vi "configure operation.vi"(7 "EthernetIP configuration":refnum<class "EthernetIP configuration.lvclass">, 8 "error in":errorcluster, 10 "line item in":T1, 11 "engine configuration in":refnum<class "engine configuration.lvclass">) -> (0 "error out":errorcluster, 1 "success":bool, 2 "line item out":T1, 5 "changed":bool)   [LabVIEW 2013, in "EthernetIP editor node.lvclass"]
uses:
  EthernetIP editor node.lvclass
  table line.ctl
  <vilib>/NI/TBM Modules/Ethernet IP/channel/EthernetIP Channel.lvclass
  <vilib>/NI/Module Execution Interface/Engine Configuration/engine configuration.lvclass
  <vilib>/NI/TBM Modules/Ethernet IP/configuration/EthernetIP configuration.lvclass
  <vilib>/NI/TBM Modules/Ethernet IP/configuration/EthernetIP configuration.lvclass/EthernetIP configuration.ctl
  <vilib>/NI/Tag Bus Module Framework/root configuration/TBM configuration.lvclass/TBM configuration.ctl
  <vilib>/NI/Tag Bus/tag/tag descriptor.lvclass/tag descriptor.ctl
  <vilib>/NI/TBM Modules/Ethernet IP/channel/EthernetIP Channel.lvclass/EthernetIP Channel.ctl
  <vilib>/NI/Tag Bus/tag/Data Type.ctl
  <vilib>/NI/Tag Bus Module Framework/channel/TBM channel.lvclass/TBM channel.ctl
  <vilib>/NI/TBM Modules/Ethernet IP/configuration/Read assemblies.vi
  <vilib>/NI/Tag Bus Module Framework/root configuration/Read instance name.vi
  <vilib>/NI/Tag Bus Module Framework/channel/Read channel classification.vi
  <vilib>/NI/Tag Bus/tag/read tag name.vi
  <vilib>/NI/Tag Bus/tag/read data type.vi
  <vilib>/NI/TBM Modules/Ethernet IP/channel/Read byte index.vi
  <vilib>/NI/TBM Modules/Ethernet IP/channel/Read subindex.vi
  <vilib>/NI/TBM Modules/Ethernet IP/channel/Read Instance ID.vi
  <vilib>/NI/Tag Bus/tag/write tag name.vi
  <vilib>/NI/Tag Bus/tag/write data type.vi
  <vilib>/NI/TBM Modules/Ethernet IP/channel/Write Instance ID.vi
  <vilib>/NI/Tag Bus Module Framework/channel/Write channel classification.vi
  <vilib>/NI/TBM Modules/Ethernet IP/channel/Write byte index.vi
  <vilib>/NI/TBM Modules/Ethernet IP/channel/Write subindex.vi
  <vilib>/NI/Tag Bus Module Framework/root configuration/create GUID.vi
  <vilib>/NI/Tag Bus/tag/tag descriptor.lvclass
panel:
  in  "refresh tags":bool
  in  "Tag":i32(listbox)
  in  "Type":i32(listbox)
  in  "Instance":i32(listbox)
  out "problem":string
  in  "subindex":i32 min=0 max=7 step=1
  in  "byte index":i32
  in  "Channel Name":string
  in  "cancel":bool
  in  "ok":bool
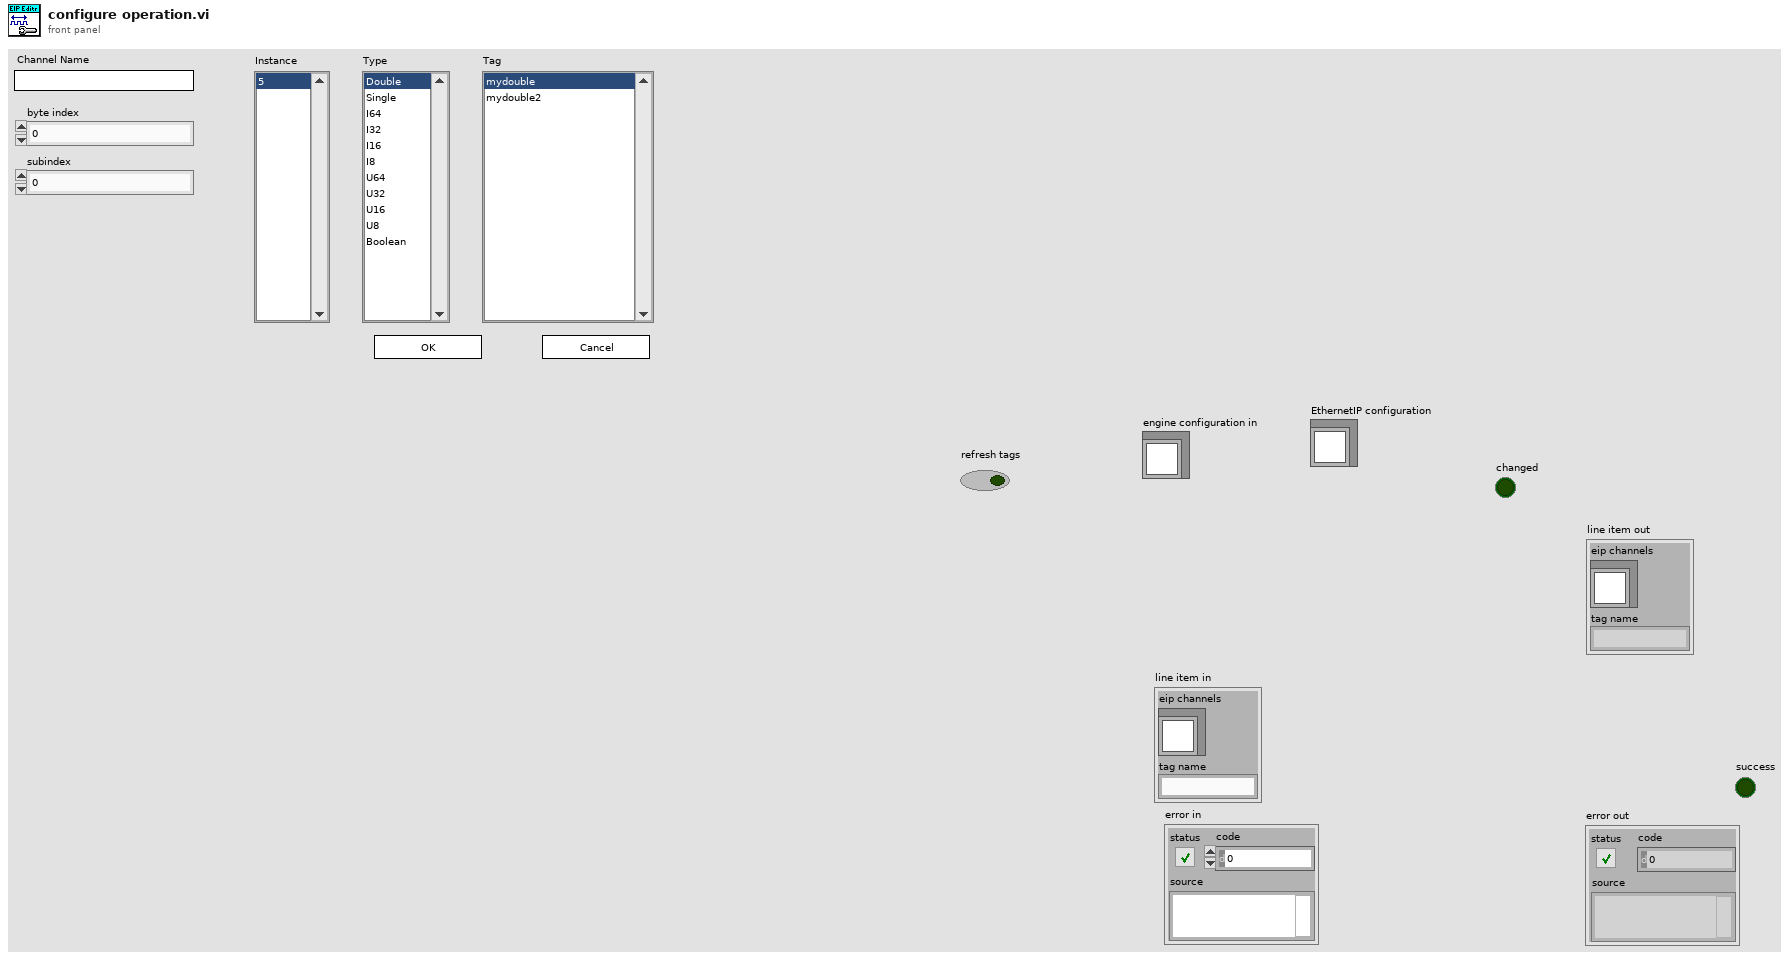
[diagram p1: front panel]
types:
  T1 = typedef "EthernetIP editor node.lvclass/table line.ctl" = cluster{"eip channels":refnum<class "EthernetIP Channel.lvclass">, "tag name":string}
  T2 = enum32{"Invalid", "Standard", "Closed", "Hidden", "Minimized", "Maximized"}
  T3 = enum32{"Invalid", "Default", "Floating", "Floating/Auto-Hide", "Modal"}
  T4 = enum8{"Enabled", "Disabled", "Disabled and Grayed Out"}
  T5 = typedef "tag bus.lvlib/tag descriptor.lvclass/Data Type.ctl" = enum16{"Double", "Single", "I64", "I32", "I16", "I8", "U64", "U32", "U16", "U8", "Boolean", "String", "Array of Double", "Array of Single", "Array of I64", "Array of I32", "Array of I16", "Array of I8", "Array of U64", "Array of U32", "Array of U16", "Array of U8", "Array of Boolean", "Array of String"}
  T6 = typedef "EthernetIP configuration.lvclass/assembly definition.ctl" = cluster{"name":string, "Instance ID":u32, "Type":T7, "Size (bytes)":u32}
  T7 = typedef "EthernetIP configuration.lvclass/assembly type.ctl" = enum32{"Producing", "Consuming"}
  T8 = enum32{"invalid app kind", "Development System", "Run Time System", "Student Edition", "Embedded LabVIEW", "Evaluation", "Custom"}
  T9 = typedef "TBM channel.lvclass/channel classification.ctl" = enum16{"input data", "output data", "processing parameter", "processing result"}
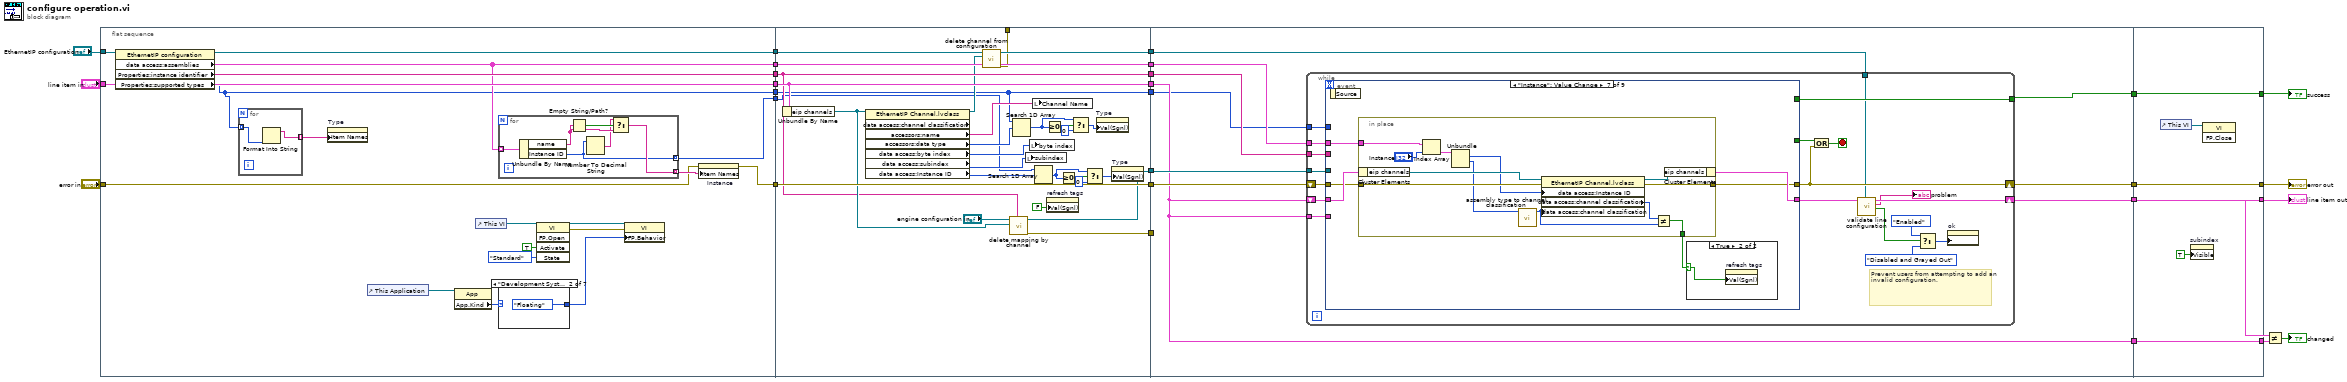
[diagram p0: block diagram]
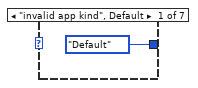
[diagram p2: hidden frame]
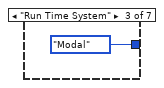
[diagram p3: hidden frame]
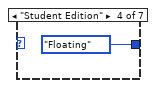
[diagram p4: hidden frame]
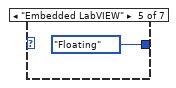
[diagram p5: hidden frame]
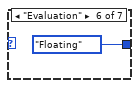
[diagram p6: hidden frame]
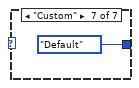
[diagram p7: hidden frame]
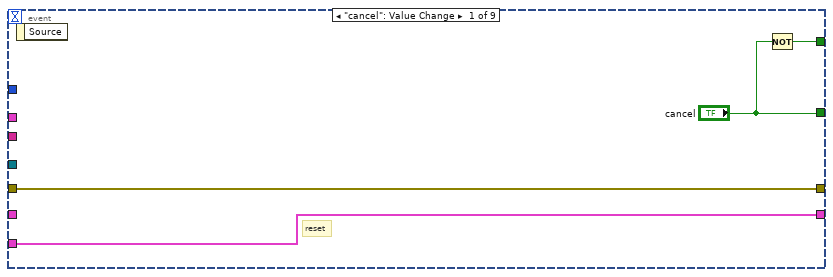
[diagram p8: hidden frame]
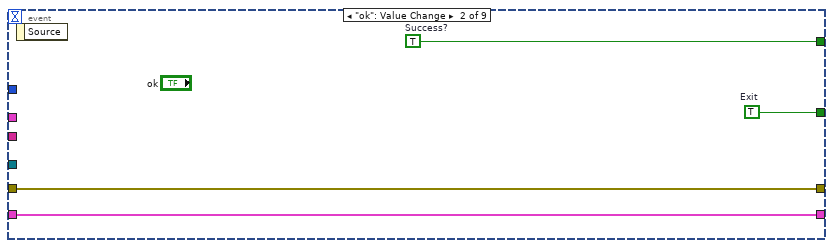
[diagram p9: hidden frame]
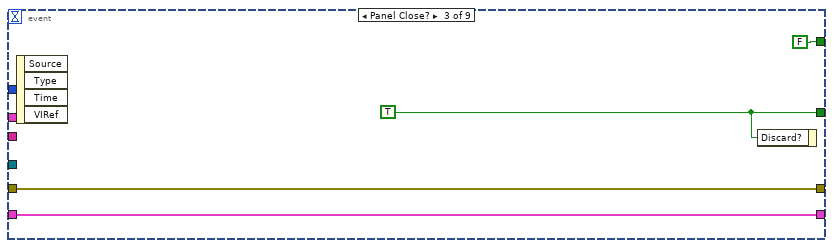
[diagram p10: hidden frame]
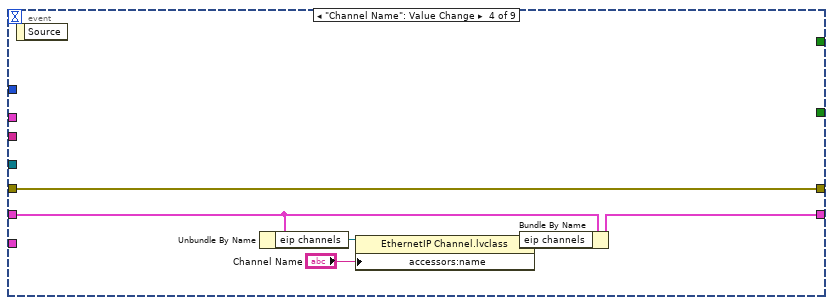
[diagram p11: hidden frame]
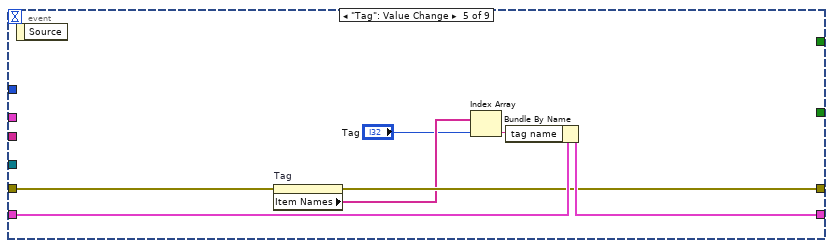
[diagram p12: hidden frame]
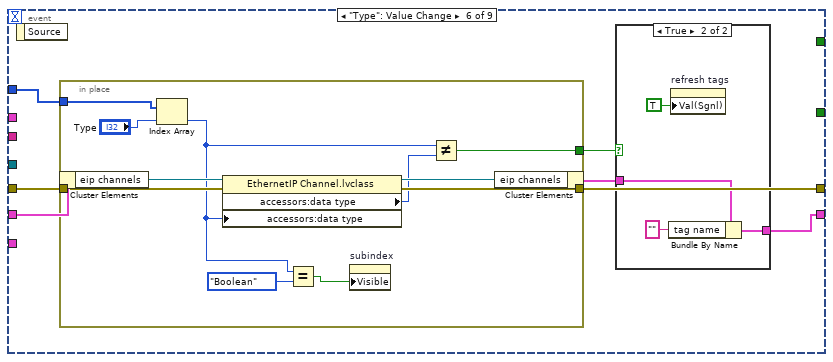
[diagram p13: hidden frame]
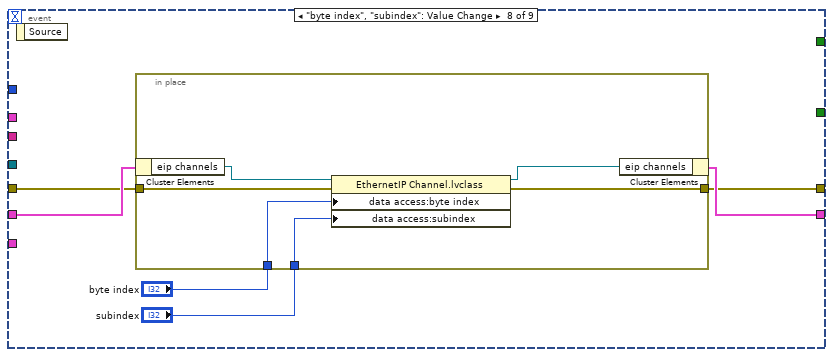
[diagram p16: hidden frame]
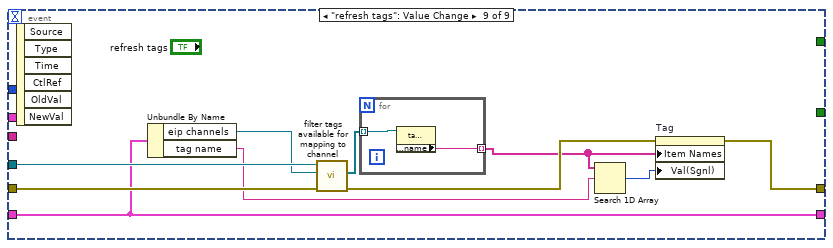
[diagram p17: hidden frame]
diagram:
  n1 = flat-sequence {
    tunnel: "line item in" -> [w46]
    tunnel: "error in" -> [w32]
    tunnel: [w31] -> w16
    tunnel: [w46] -> w14
    tunnel: "EthernetIP configuration" -> [w37]
    tunnel: [w36] -> w8
    tunnel: [w34] -> w6
    tunnel: [w35] -> w5
    tunnel: [w30] -> w2
    tunnel: [w28] -> w1
    tunnel: w16 -> [w89]
    tunnel: [w89] -> w15
    tunnel: w14 -> [w87]
    tunnel: [w87] -> w13
    tunnel: [w85] -> w12
    tunnel: [w84] -> w11
    tunnel: [w77] -> w9
    tunnel: w8 -> [w80]
    tunnel: [w79] -> w7
    tunnel: w6 -> [w79]
    tunnel: w5 -> [w78]
    tunnel: [w78] -> w4
    tunnel: [w75] -> _
    tunnel: [w74] -> w3
    tunnel: w2 -> [w74]
    tunnel: w1 -> [w68]
    tunnel: [w98] -> w20
    tunnel: [w97] -> w19
    tunnel: [w96] -> w18
    tunnel: [w91] -> w17
    tunnel: w15 -> [w99]
    tunnel: w13 -> [w91]
    tunnel: w12 -> [_]
    tunnel: w11 -> [w95]
    tunnel: w9 -> [w94]
    tunnel: w7 -> [w93]
    tunnel: w4 -> [w92]
    tunnel: w3 -> [w90]
    tunnel: [w211] -> w21
    tunnel: [w212] -> w24
    tunnel: [w213] -> w25
    tunnel: [w214] -> w26
    tunnel: w20 -> [w214]
    tunnel: w19 -> [w213]
    tunnel: w18 -> [w212]
    tunnel: w17 -> [w211]
    frame #0 {
      n2 = property class="EthernetIP configuration"(reference=w37) -> (reference out=w36:refnum<class "EthernetIP configuration.lvclass">, "data access:assemblies"=w34:T6[], "Properties:instance identifier"=w35:string, "Properties:supported types"=w30:T5[])  [unwired: 1 in, 1 out]
      n3 = for {
        tunnel: w30 -> [w48] mode=indexing
        tunnel: [w47] -> w29 mode=indexing
        n4 = Format Into String(w48) -> (resulting string=w47:string)  [unwired: 3 in, 1 out]
      }
      n5 = property on="Type" class="LstBox (strict)"("Item Names"=w29) -> ()  [unwired: 2 in, 2 out]
      n6 = control-ref of="This Application"() -> (w40:refnum<vi>)
      n7 = property class="App"(reference=w40) -> ("App.Kind"=w39:T8)  [unwired: 1 in, 2 out]
      n8 = control-ref of="This VI"() -> (w41:refnum<vi>)
      n9 = for {
        tunnel: w34 -> [w54] mode=indexing
        tunnel: [w50] -> w33 mode=indexing
        tunnel: [w49] -> w28 mode=indexing
        n10 = Unbundle By Name(w54) -> ("name"=w52:string, "Instance ID"=w49:u32)
        n11 = Empty String/Path?(string/path=w52) -> (empty?=w53:bool)
        n12 = Number To Decimal String(number=w49) -> (decimal integer string=w51:string)  [unwired: 1 in]
        n13 = Select(t=w51, s=w53, f=w52) -> (s? t:f=w50:string)
      }
      n14 = case shown="\"Development System\"" w39 {
        tunnel: [T3."Default" ("Front Panel Window:Behavior") T3."Floating" ("Front Panel Window:Behavior") T3."Modal" ("Front Panel Window:Behavior") T3."Floating" ("Front Panel Window:Behavior") T3."Floating" ("Front Panel Window:Behavior") T3."Floating" ("Front Panel Window:Behavior") T3."Default" ("Front Panel Window:Behavior")] -> w38
        frame "invalid app kind", Default {
        }
        frame "Development System" {
        }
        frame "Run Time System" {
        }
        frame "Student Edition" {
        }
        frame "Embedded LabVIEW" {
        }
        frame "Evaluation" {
        }
        frame "Custom" {
        }
      }
      n15 = invoke class="VI" method="FP.Open"(reference=w41, "Activate"=TRUE ("Activate?"), "State"=T2."Standard") -> (reference out=w44:refnum<vi>, error out=w45:errorcluster)  [unwired: 2 in, 3 out]
      n16 = property class="VI"(reference=w44, error in=w45, "FP.Behavior"=w38) -> ()  [unwired: 2 out]
      n17 = property on="Instance" class="LstBox (strict)"(error in=w32, "Item Names"=w33) -> (error out=w31:errorcluster)  [unwired: 1 in, 1 out]
    }
    frame #1 {
      n18 = Unbundle By Name(w87) -> ("eip channels"=w83:refnum<class "EthernetIP Channel.lvclass">)
      n19 = property class="EthernetIP Channel.lvclass" props=["data access:channel classification", "accessors:name", "accessors:data type", "data access:byte index", "data access:subindex", "data access:Instance ID"](reference=w83) -> (reference out=w76:refnum<class "EthernetIP Channel.lvclass">, "accessors:name"=w88:string, "accessors:data type"=w73:T5, "data access:byte index"=w82:i32, "data access:subindex"=w81:i32, "data access:Instance ID"=w63:u32)  [unwired: 1 in, 2 out]
      n20 = call <vilib>:"delete channel from configuration.vi"("TBM channel in"=w76, "EthernetIP configuration in"=w80) -> ("error out"=w75:errorcluster, "EthernetIP configuration out"=w77:refnum<class "EthernetIP configuration.lvclass">)  [unwired: 8 in]
      n21 = call <vilib>:"delete mapping by channel.vi"("owner ID"=w78, "channel"=w83, "engine configuration in"="engine configuration in") -> ("error out"=w85:errorcluster, "engine configuration out"=w84:refnum<class "engine configuration.lvclass">)  [unwired: 7 in]
      n22 = Search 1D Array(1D array=w74, element=w73) -> (index of element=w71:i32)  [unwired: 1 in]
      n23 = local write "subindex"(w81) -> ()
      n24 = local write "byte index"(w82) -> ()
      n25 = local write "Channel Name"(w88) -> ()
      n26 = Search 1D Array(1D array=w68, element=w63) -> (index of element=w65:i32)  [unwired: 1 in]
      n27 = Greater Or Equal To 0?(x=w71) -> (x >= 0?=w72:bool)
      n28 = property on="refresh tags" class="Bool (strict)"("Val(Sgnl)"=FALSE ("Value (Signaling)")) -> ()  [unwired: 2 in, 2 out]
      n29 = Greater Or Equal To 0?(x=w65) -> (x >= 0?=w66:bool)
      n30 = Select(t=w71, s=w72, f=0) -> (s? t:f=w69:i32)
      n31 = Select(t=w65, s=w66, f=0) -> (s? t:f=w64:i32)
      n32 = property on="Type" class="LstBox (strict)"("Val(Sgnl)"=w69) -> ()  [unwired: 2 in, 2 out]
      n33 = property on="Type" class="LstBox (strict)"("Val(Sgnl)"=w64) -> ()  [unwired: 2 in, 2 out]
    }
    frame #2 {
      n34 = while {
        shift-right: [w109] -> w97
        shift-left: w99 -> [w117]
        tunnel: [w116] -> w98
        shift-right: [w110] -> w96
        shift-left: w91 -> [w113]
        tunnel: w91 -> [w112]
        tunnel: w95 -> [w118]
        tunnel: w94 -> [w104]
        tunnel: w93 -> [w103]
        tunnel: w92 -> [w102]
        tunnel: w90 -> [w100]
        stop <- w114 stop-if-true
        # "Prevent users from attempting to add an invalid configuration."
        n35 = event shown="[6] \"Instance\": Value Change" {
          selector: _ -> [_ _ _ _ _ _ _ _ _]
          dyn-events: _ -> [_ _ _ _ _ _ _ _ _]
          timeout: _ -> [_ _ _ _ _ _ _ _ _]
          tunnel: w118 -> [_ _ _ _ _ _ _ _ w204]
          tunnel: w117 -> [w122 w126 w130 w136 w142 w149 w170 w189 w206]
          tunnel: [w122 w126 w130 w136 w139 w148 w169 w188 w205] -> w109
          tunnel: [w121 w123 FALSE _ _ _ _ _ _] -> w116
          tunnel: ["cancel" w124 w128 _ _ _ _ _ _] -> w115
          tunnel: w113 -> [_ w125 w127 w134 w143 w150 w172 w191 w203]
          tunnel: [w119 w125 w127 w135 w141 w145 w171 w190 w203] -> w111
          tunnel: w112 -> [w119 _ _ _ _ _ _ _ _]
          tunnel: w103 -> [_ _ _ _ _ _ w167 _ _]
          tunnel: w102 -> [_ _ _ _ _ _ _ _ _]
          tunnel: w100 -> [_ _ _ _ _ w144 _ _ _]
          event "cancel": Value Change {
            # "reset"
            n36 = event-data() -> ()  [unwired: 1 in, 1 out]
            n37 = Not(x="cancel") -> (.not. x?=w121:bool)
          }
          event "ok": Value Change {
            w123 = TRUE  # Success?
            w124 = TRUE  # Exit
            n38 = event-data() -> ()  [unwired: 1 in, 1 out]
          }
          event Panel Close? {
            w128 = TRUE ("cancel")
            n39 = event-data() -> ()  [unwired: 1 in, 4 out]
            n40 = event-data("Discard?"=w128) -> ()  [unwired: 1 in, 1 out]
          }
          event "Channel Name": Value Change {
            n41 = event-data() -> ()  [unwired: 1 in, 1 out]
            n42 = Unbundle By Name(w134) -> ("eip channels"=w133:refnum<class "EthernetIP Channel.lvclass">)
            n43 = property class="EthernetIP Channel.lvclass"(reference=w133, "accessors:name"="Channel Name") -> (reference out=w132:refnum<class "EthernetIP Channel.lvclass">)  [unwired: 1 in, 1 out]
            n44 = Bundle By Name(cluster=w134, "eip channels"=w132) -> (w135:T1)
          }
          event "Tag": Value Change {
            n45 = event-data() -> ()  [unwired: 1 in, 1 out]
            n46 = property on="Tag" class="LstBox (strict)"(error in=w142) -> (error out=w139:errorcluster, "Item Names"=w138:string[])  [unwired: 1 in, 1 out]
            n47 = Index Array(array=w138, index="Tag") -> (element=w140:string)
            n48 = Bundle By Name(cluster=w143, "tag name"=w140) -> (w141:T1)
          }
          event "Type": Value Change {
            n49 = event-data() -> ()  [unwired: 1 in, 1 out]
            n50 = in-place {
              in-place-border: w149 -> [w165]
              in-place-border: [w164] -> w148
              in-place-border: [w159] -> w147
              in-place-border: w144 -> [w158]
              n51 = in-place-cluster #1(w150) -> ("eip channels"=w166:refnum<class "EthernetIP Channel.lvclass">)
              n52 = Index Array(array=w158, index="Type") -> (element=w156:T5)
              n53 = property class="EthernetIP Channel.lvclass"(reference=w166, error in=w165, "accessors:data type"=w156) -> (reference out=w163:refnum<class "EthernetIP Channel.lvclass">, error out=w164:errorcluster, "accessors:data type"=w160:T5)
              n54 = Equal?(x=w156, y=Data_Type."Boolean") -> (x = y?=w161:bool)
              n55 = property on="subindex" class="DigNum (strict)"("Visible"=w161) -> ()  [unwired: 2 in, 2 out]
              n56 = Not Equal?(x=w156, y=w160) -> (x != y?=w159:bool)
              n57 = in-place-cluster #1("eip channels"=w163) -> (w146:T1)
            }
            n58 = case shown="True" w147 {
              tunnel: w146 -> [w151 w154]
              tunnel: [w151 w153] -> w145
              frame False {
              }
              frame True {
                n59 = Bundle By Name(cluster=w154, "tag name"="") -> (w153:T1)
                n60 = property on="refresh tags" class="Bool (strict)"("Val(Sgnl)"=TRUE ("Value (Signaling)")) -> ()  [unwired: 2 in, 2 out]
              }
            }
          }
          event "Instance": Value Change {
            n61 = event-data() -> ()  [unwired: 1 in, 1 out]
            n62 = in-place {
              in-place-border: w170 -> [w185]
              in-place-border: [w184] -> w169
              in-place-border: [w179] -> w168
              in-place-border: w167 -> [w177]
              n63 = in-place-cluster #2(w172) -> ("eip channels"=w183:refnum<class "EthernetIP Channel.lvclass">)
              n64 = Index Array(array=w177, index="Instance") -> (element=w176:T6)
              n65 = Unbundle(w176) -> ("Instance ID"=w175:u32, "Type"=w174:T7)  [unwired: 2 out]
              n66 = call <vilib>:"assembly type to channel classification.vi"("Type"=w174) -> ("channel classification"=w180:T9)  [unwired: 10 in]
              n67 = property class="EthernetIP Channel.lvclass"(reference=w183, error in=w185, "data access:Instance ID"=w175, "data access:channel classification"=w180) -> (reference out=w182:refnum<class "EthernetIP Channel.lvclass">, error out=w184:errorcluster, "data access:channel classification"=w181:T9)
              n68 = Not Equal?(x=w181, y=w180) -> (x != y?=w179:bool)
              n69 = in-place-cluster #2("eip channels"=w182) -> (w171:T1)
            }
            n70 = case shown="True" w168 {
              selector: w168 -> [_ w173]
              frame False {
              }
              frame True {
                n71 = property on="refresh tags" class="Bool (strict)"("Val(Sgnl)"=w173) -> ()  [unwired: 2 in, 2 out]
              }
            }
          }
          event "byte index", "subindex": Value Change {
            n72 = event-data() -> ()  [unwired: 1 in, 1 out]
            n73 = in-place {
              in-place-border: w189 -> [w197]
              in-place-border: [w196] -> w188
              in-place-border: "subindex" -> [w193]
              in-place-border: "byte index" -> [w192]
              n74 = in-place-cluster #3(w191) -> ("eip channels"=w195:refnum<class "EthernetIP Channel.lvclass">)
              n75 = property class="EthernetIP Channel.lvclass"(reference=w195, error in=w197, "data access:byte index"=w192, "data access:subindex"=w193) -> (reference out=w194:refnum<class "EthernetIP Channel.lvclass">, error out=w196:errorcluster)
              n76 = in-place-cluster #3("eip channels"=w194) -> (w190:T1)
            }
          }
          event "refresh tags": Value Change {
            n77 = event-data() -> ()  [unwired: 1 in, 6 out]
            n78 = Unbundle By Name(w203) -> ("eip channels"=w202:refnum<class "EthernetIP Channel.lvclass">, "tag name"=w199:string)
            n79 = call <vilib>:"filter tags available for mapping to channel.vi"("channel to map to"=w202, "engine configuration in"=w204) -> ("filtered tags"=w201:refnum<class "tag descriptor.lvclass">[])  [unwired: 8 in, 1 out]
            n80 = for {
              tunnel: w201 -> [w208] mode=indexing
              tunnel: [w207] -> w200 mode=indexing
              n81 = property class="tag descriptor"(reference=w208) -> ("accessors:name"=w207:string)  [unwired: 1 in, 2 out]
            }
            n82 = Search 1D Array(1D array=w200, element=w199) -> (index of element=w198:i32)  [unwired: 1 in]
            n83 = property on="Tag" class="LstBox (strict)"(error in=w206, "Item Names"=w200, "Val(Sgnl)"=w198) -> (error out=w205:errorcluster)  [unwired: 1 in, 1 out]
          }
        }
        n84 = Compound Arithmetic op=OR(w115, w109) -> (w114:bool)
        n85 = call "validate line configuration.vi"("EthernetIP configuration"=w104, "line in"=w111) -> ("valid?"=w108:bool, "problem"=→"problem":string, "line out"=w110:T1)  [unwired: 7 in]
        n86 = Select(t=T4."Enabled" ("Disabled"), s=w108, f=T4."Disabled and Grayed Out") -> (s? t:f=w105:T4)
        n87 = property on="ok" class="Bool"("DisabledEnum"=w105) -> ()  [unwired: 2 in, 2 out]
      }
    }
    frame #3 {
      n88 = control-ref of="This VI"() -> (w210:refnum<vi>)
      n89 = property on="subindex" class="DigNum (strict)"("Visible"=TRUE) -> ()  [unwired: 2 in, 2 out]
      n90 = invoke class="VI" method="FP.Close"(reference=w210) -> ()  [unwired: 2 in, 3 out]
    }
  }
  n91 = Not Equal?(x=w24, y=w21) -> (x != y?=→"changed":bool)
  "error out" <- w25
  "success" <- w26
  "line item out" <- w24
